vi "配置控件.vi"(4 "原备注":string, 5 "交互信息":string, 6 "关键字":string, 7 "原值":string) -> (0 "新备注":string, 1 "新值":string)   [LabVIEW 2018]
panel:
  in  "备注":string
  in  "确定":bool
  in  "取消":bool
  in  "选项卡":enum32{"for", "in", "out", "compare", "logic"}(tab)
  in  "列表":string
  in  "元素":string
  in  "变量/常量":string
  in  "提示":u16(ring) items=["LED灯序号", "状态"]
  in  "备选信息":u16(ring) items=["", "on"]
  in  "out":string
  in  "比较符号":enum16{"", "==", "!=", ">", "<", ">=", "<="}(ring)
  in  "逻辑运算":enum16{"", "and", "or", "not"}(ring)
  # "："
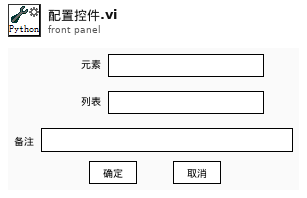
[diagram p1: front panel]
types:
  T1 = typedef "eventvkey.ctl" = enum16{"ASCII", "Enter", "Return", "Shift", "Ctrl", "Alt", "Cmd", "Opt", "Caps", "NumLock", "Clear", "Break", "Up", "Down", "Left", "Right", "Insert", "Delete", "Home", "End", "PageUp", "PageDown", "Escape", "Help", "Pause", "ScrollLock", "F1", "F2", "F3", "F4", "F5", "F6", "F7", "F8", "F9", "F10", "F11", "F12", "F13", "F14", "F15", "F16", "F17", "F18", "F19", "F20", "F21", "F22", "F23", "F24", "Play", "VolumeUp", "VolumeDown", "Mute", "Two Byte Char"}
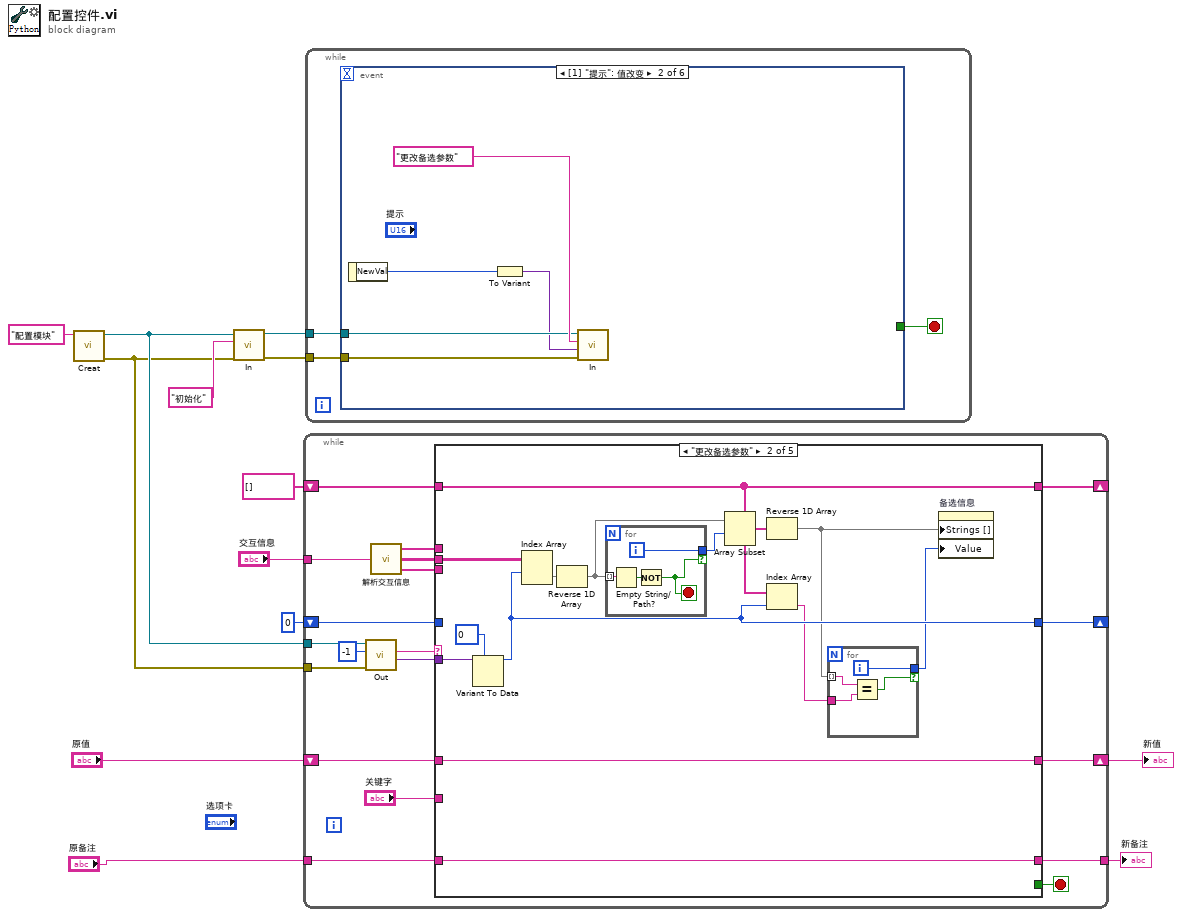
[diagram p0: block diagram]
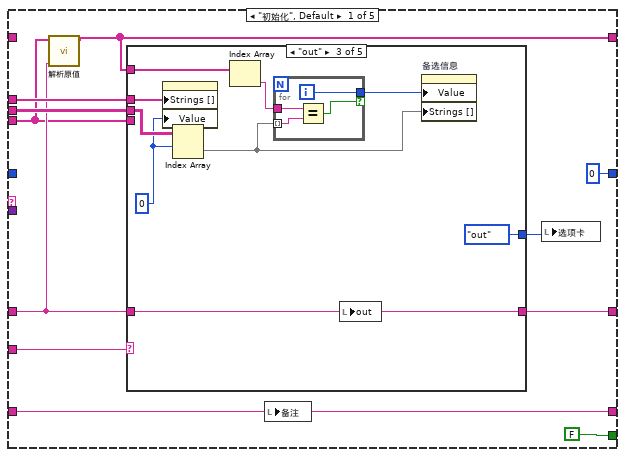
[diagram p2: hidden frame]
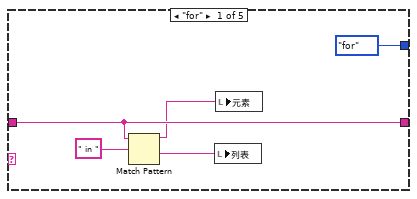
[diagram p3: hidden frame]
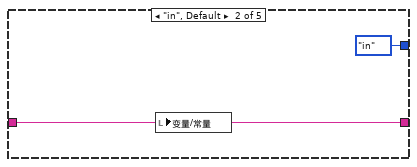
[diagram p4: hidden frame]
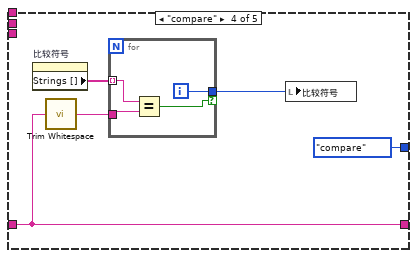
[diagram p5: hidden frame]
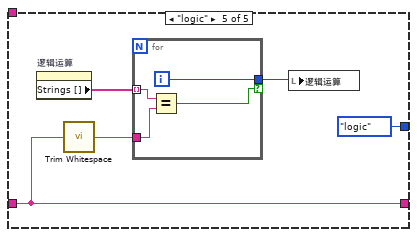
[diagram p6: hidden frame]
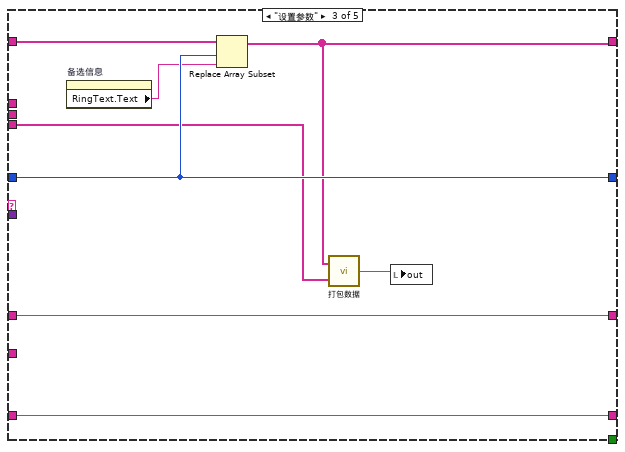
[diagram p7: hidden frame]
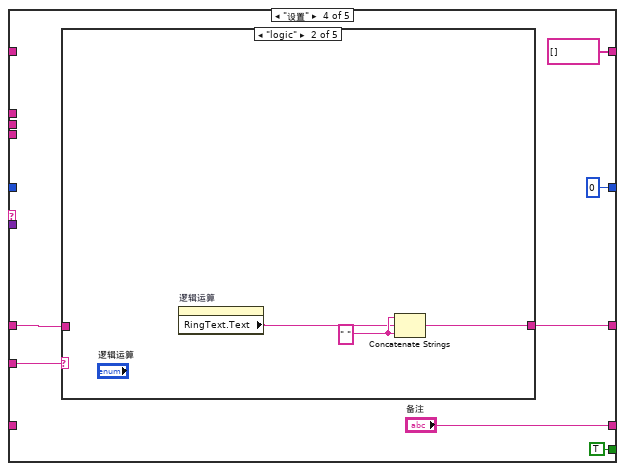
[diagram p8: hidden frame]
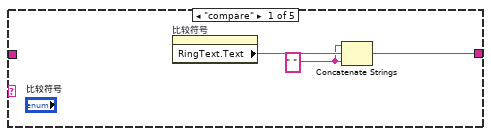
[diagram p9: hidden frame]
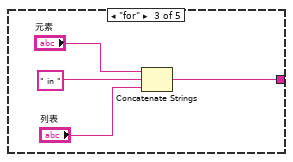
[diagram p10: hidden frame]
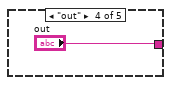
[diagram p11: hidden frame]
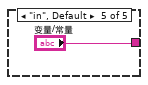
[diagram p12: hidden frame]
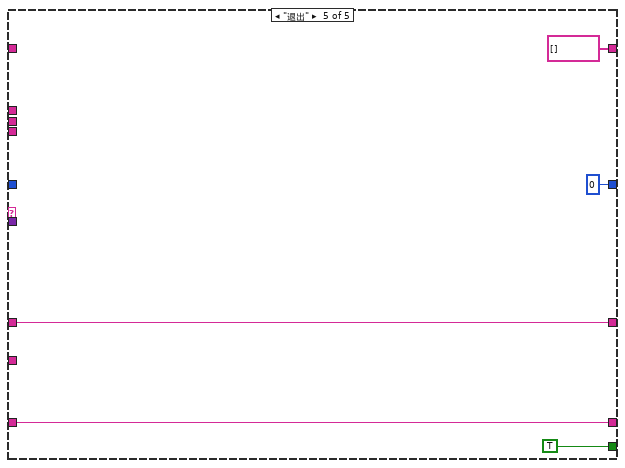
[diagram p13: hidden frame]
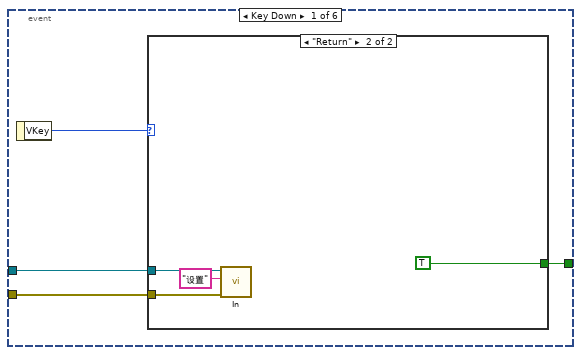
[diagram p14: hidden frame]
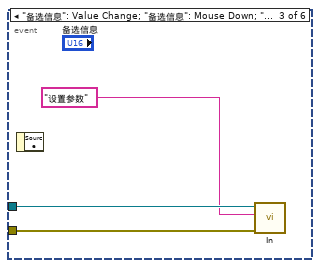
[diagram p16: hidden frame]
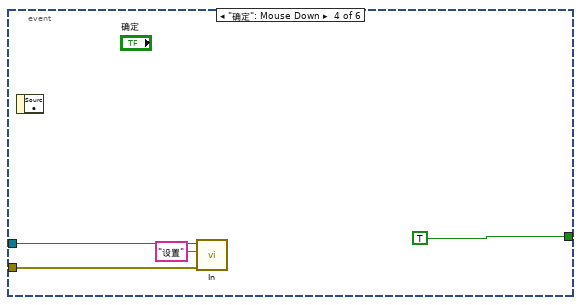
[diagram p17: hidden frame]
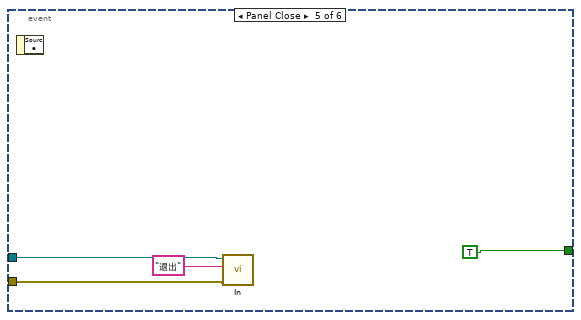
[diagram p18: hidden frame]
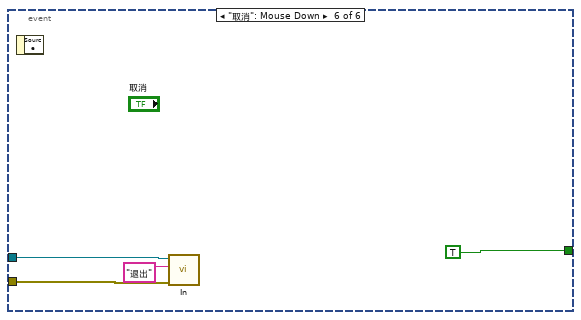
[diagram p19: hidden frame]
diagram:
  n1 = call "Creat.vi"("名称"="配置模块") -> ("错误输出"=w6:errorcluster, "队列输出"=w7:refnum<queue>)  [unwired: 9 in]
  n2 = call "In.vi"("错误输入"=w6, "指令"="初始化", "队列"=w7) -> ("错误输出"=w9:errorcluster, "队列输出"=w8:refnum<queue>)  [unwired: 7 in]
  n3 = while {
    shift-right: [w31] -> w11
    shift-left: "原值" -> [w32]
    tunnel: w7 -> [w28]
    tunnel: w6 -> [w27]
    tunnel: "交互信息" -> [w23]
    shift-right: [w19] -> _
    shift-left: string[] [] ("提示") -> [w18]
    shift-right: [w17] -> _
    shift-left: u16 0 ("提示") -> [w16]
    tunnel: [w15] -> w1
    tunnel: "原备注" -> [w14]
    stop <- w30 stop-if-true
    n4 = call "Out.vi"("错误输入"=w27, "超时毫秒(-1)"=-1, "队列"=w28) -> ("数据"=w24:variant, "指令"=w26:string)  [unwired: 5 in, 2 out]
    n5 = call "解析交互信息.vi"("交互信息"=w23) -> ("提示"=w22:string[], "备选信息"=w21:string[][], "补充信息"=w20:string[])  [unwired: 4 in]
    n6 = case shown="\"更改备选参数\"" w26 {
      tunnel: w32 -> [w37 w93 w109 w115 w132]
      tunnel: "关键字" -> [w43 _ _ w118 _]
      tunnel: [w42 w93 w109 w117 w132] -> w31
      tunnel: [FALSE _ _ TRUE TRUE] -> w30
      tunnel: w24 -> [_ w95 _ _ _]
      tunnel: w22 -> [w39 _ _ _ _]
      tunnel: w21 -> [w40 w94 _ _ _]
      tunnel: w20 -> [w36 _ w107 _ _]
      tunnel: [w35 w91 w108 string[] [] ("提示") string[] [] ("提示")] -> w19
      tunnel: w18 -> [_ w91 w111 _ _]
      tunnel: [u16 0 ("提示") w90 w110 u16 0 ("提示") u16 0 ("提示")] -> w17
      tunnel: w16 -> [_ _ w110 _ _]
      tunnel: [w34 w87 w104 "备注" w131] -> w15
      tunnel: w14 -> [w34 w87 w104 _ w131]
      frame "初始化", Default {
        n7 = call "解析原值.vi"("原值"=w37, "补充信息"=w36) -> ("参数"=w35:string[])  [unwired: 9 in]
        n8 = case shown="\"out\"" w43 {
          tunnel: w37 -> [w48 w50 w58 w67 w77]
          tunnel: [w48 w50 w58 w67 w77] -> w42
          tunnel: w39 -> [_ _ w59 _ _]
          tunnel: w40 -> [_ _ w57 _ _]
          tunnel: w36 -> [_ _ _ _ _]
          tunnel: w35 -> [_ _ w54 _ _]
          tunnel: [enum32{"for", "in", "out", "compare", "logic"}."for" ("选项卡") enum32{"for", "in", "out", "compare", "logic"}."in" ("选项卡") enum32{"for", "in", "out", "compare", "logic"}."out" ("选项卡") enum32{"for", "in", "out", "compare", "logic"}."compare" ("选项卡") enum32{"for", "in", "out", "compare", "logic"}."logic" ("选项卡")] -> w33
          frame "for" {
            n9 = Match Pattern(string=w48, regular expression=" in " ("字符串")) -> (before substring=w47:string, after substring=w46:string)  [unwired: 1 in, 2 out]
            n10 = local write "列表"(w46) -> ()
            n11 = local write "元素"(w47) -> ()
          }
          frame "in", Default {
            n12 = local write "变量/常量"(w50) -> ()
          }
          frame "out" {
            w56 = u16 0
            n13 = property on="提示" class="Ring (严格)"("Strings []"=w59, "Value"=w56) -> ()  [unwired: 2 in, 2 out]
            n14 = Index Array(array=w57, index (row)=w56) -> (element=w52:string[])  [unwired: 1 in]
            n15 = Index Array(array=w54) -> (element=w53:string)  [unwired: 1 in]
            n16 = for {
              tunnel: w53 -> [w62]
              tunnel: w52 -> [w63] mode=indexing
              tunnel: [w61] -> w55 if=w60
              i -> [w61]
              n17 = Equal?(x=w62, y=w63) -> (x = y?=w60:bool)
            }
            n18 = local write "out"(w58) -> ()
            n19 = property on="备选信息" class="Ring (严格)"("Value"=w55, "Strings []"=w52) -> ()  [unwired: 2 in, 2 out]
          }
          frame "compare" {
            n20 = property on="比较符号" class="Enum (严格)"() -> ("Strings []"=w68:string[])  [unwired: 2 in, 2 out]
            n21 = call <vilib>:"Trim Whitespace.vi"("string"=w67) -> ("trimmed string"=w65:string)  [unwired: 1 in]
            n22 = for {
              tunnel: w65 -> [w70]
              tunnel: [w72] -> w66 if=w69
              tunnel: w68 -> [w71] mode=indexing
              i -> [w72]
              n23 = Equal?(x=w71, y=w70) -> (x = y?=w69:bool)
            }
            n24 = local write "比较符号"(w66) -> ()
          }
          frame "logic" {
            n25 = property on="逻辑运算" class="Enum (严格)"() -> ("Strings []"=w76:string[])  [unwired: 2 in, 2 out]
            n26 = call <vilib>:"Trim Whitespace.vi"("string"=w77) -> ("trimmed string"=w74:string)  [unwired: 1 in]
            n27 = for {
              tunnel: w74 -> [w81]
              tunnel: w76 -> [w80] mode=indexing
              tunnel: [w79] -> w75 if=w78
              i -> [w79]
              n28 = Equal?(x=w80, y=w81) -> (x = y?=w78:bool)
            }
            n29 = local write "逻辑运算"(w75) -> ()
          }
        }
        n30 = local write "备注"(w34) -> ()
        n31 = local write "选项卡"(w33) -> ()
      }
      frame "更改备选参数" {
        w92 = u16 0 items=[""] ("提示")
        n32 = Variant To Data(type=w92, Variant=w95) -> (data=w90:u16)  [unwired: 1 in, 1 out]
        n33 = Index Array(array=w94, index (row)=w90) -> (element=w86:string[])  [unwired: 1 in]
        n34 = Reverse 1D Array(array=w86) -> (reversed array=w85:string[])
        n35 = for {
          tunnel: w85 -> [w99] mode=indexing
          tunnel: [w98] -> w84 if=w96
          i -> [w98]
          stop <- w96 stop-if-true
          n36 = Empty String/Path?(string/path=w99) -> (empty?=w97:bool)
          n37 = Not(x=w97) -> (.not. x?=w96:bool)
        }
        n38 = Array Subset(array=w85, index=w84) -> (w83:string[])  [unwired: 1 in]
        n39 = Reverse 1D Array(array=w83) -> (reversed array=w82:string[])
        n40 = Index Array(array=w91, index=w90) -> (element=w89:string)
        n41 = for {
          tunnel: w89 -> [w102]
          tunnel: w82 -> [w103] mode=indexing
          tunnel: [w101] -> w88 if=w100
          i -> [w101]
          n42 = Equal?(x=w103, y=w102) -> (x = y?=w100:bool)
        }
        n43 = property on="备选信息" class="Ring (严格)"("Strings []"=w82, "Value"=w88) -> ()  [unwired: 2 in, 2 out]
      }
      frame "设置参数" {
        n44 = property on="备选信息" class="Ring (严格)"() -> ("RingText.Text"=w105:string)  [unwired: 2 in, 2 out]
        n45 = Replace Array Subset(array=w111, new element=w105, index=w110) -> (w108:string[])
        n46 = call "打包数据.vi"("补充信息"=w107, "备选信息"=w108) -> ("语句"=w106:string)
        n47 = local write "out"(w106) -> ()
      }
      frame "设置" {
        n48 = case shown="\"logic\"" w118 {
          tunnel: [w120 w124 w125 "out" "变量/常量"] -> w117
          tunnel: w115 -> [_ _ _ _ _]
          frame "compare" {
            w119 = " " ("字符串")
            n49 = property on="比较符号" class="Enum (严格)"() -> ("RingText.Text"=w121:string)  [unwired: 2 in, 2 out]
            n50 = Concatenate Strings(w119, w121, w119) -> (w120:string)
          }
          frame "logic" {
            w123 = " " ("字符串")
            n51 = property on="逻辑运算" class="Enum (严格)"() -> ("RingText.Text"=w122:string)  [unwired: 2 in, 2 out]
            n52 = Concatenate Strings(w123, w122, w123) -> (w124:string)
          }
          frame "for" {
            n53 = Concatenate Strings("元素", " in " ("字符串"), "列表") -> (w125:string)
          }
          frame "out" {
          }
          frame "in", Default {
          }
        }
      }
      frame "退出" {
      }
    }
  }
  "新值" <- w11
  "新备注" <- w1
  n54 = while {
    tunnel: w8 -> [w137]
    tunnel: w9 -> [w136]
    stop <- w138 stop-if-true
    n55 = event shown="[1] \"提示\": 值改变" {
      selector: _ -> [_ _ _ _ _ _]
      dyn-events: _ -> [_ _ _ _ _ _]
      timeout: _ -> [_ _ _ _ _ _]
      tunnel: [w141 _ _ TRUE TRUE TRUE] -> w138
      tunnel: w137 -> [w140 w150 w154 w156 w161 w164]
      tunnel: w136 -> [w139 w149 w153 w155 w159 w163]
      event Key Down {
        n56 = event-data() -> ("VKey"=w142:T1)  [unwired: 1 in]
        n57 = case shown="\"Return\"" w142 {
          tunnel: [_ TRUE] -> w141
          tunnel: w140 -> [_ w145]
          tunnel: w139 -> [_ w144]
          frame "Shift", Default {
          }
          frame "Return" {
            n58 = call "In.vi"("错误输入"=w144, "指令"="设置", "队列"=w145) -> ()  [unwired: 7 in, 2 out]
          }
        }
      }
      event "提示": Value Change {
        n59 = event-data() -> ("NewVal"=w147:u16)  [unwired: 1 in]
        n60 = To Variant(anything=w147) -> (Variant=w148:variant)
        n61 = call "In.vi"("错误输入"=w149, "数据"=w148, "指令"="更改备选参数", "队列"=w150) -> ()  [unwired: 6 in, 2 out]
      }
      event "备选信息": Value Change; "备选信息": Mouse Down; "备选信息": Mouse Up {
        n62 = event-data() -> ()  [unwired: 1 in, 1 out]
        n63 = call "In.vi"("错误输入"=w153, "指令"="设置参数", "队列"=w154) -> ()  [unwired: 7 in, 2 out]
      }
      event "确定": Mouse Down {
        n64 = event-data() -> ()  [unwired: 1 in, 1 out]
        n65 = call "In.vi"("错误输入"=w155, "指令"="设置", "队列"=w156) -> ()  [unwired: 7 in, 2 out]
      }
      event Panel Close {
        n66 = event-data() -> ()  [unwired: 1 in, 1 out]
        n67 = call "In.vi"("错误输入"=w159, "指令"="退出", "队列"=w161) -> ()  [unwired: 7 in, 2 out]
      }
      event "取消": Mouse Down {
        n68 = event-data() -> ()  [unwired: 1 in, 1 out]
        n69 = call "In.vi"("错误输入"=w163, "指令"="退出", "队列"=w164) -> ()  [unwired: 7 in, 2 out]
      }
    }
  }
